vi "NeedRecalcPath.vi"(0 "Project":T1, 1 "AttackerAvoidArea":bool=TRUE, 4 "ignoreBall?":bool, 5 "Initial State":dbl[](array[numeric]), 6 "SmoothPath":dbl[][](array[numeric]), 7 "Pos x,y":dbl[](array[numeric]), 8 "Volta ao redor\nda área?":bool, 9 "IA State":T2={"our_robots"=[], "enemy_robots"=[], "balls"=[], "geometry"={"line_width"=0, "field_length"=0, "field_width"=0, "boundary_width"=0, "referee_width"=0, "goal_width"=0, "goal_depth"=0, "goal_wall_width"=0, "center_circle_radius"=0, "defense_radius"=0, "defense_stretch"=0, "free_kick_from_defense_dist"=0, "penalty_spot_from_field_line_dist"=0, "penalty_line_from_spot_dist"=0}, "IA Judge"={"stage"="", "command"="", "our_goalie_id"=0.0, "enemy_goalie_id"=0.0, "command enum"=enum."Halt", "Time"=enum."Azul", "Point"={"x"=0.0, "y"=0.0}}, "Received Timestamp"=timestamp(0 s since 1904-01-01), "Events"={"Touch"=FALSE, "Ball out"=FALSE, "id touch"=0.0, "Ball out of \nVision"=FALSE, "Ball inside \nGoalie area"=FALSE, "Robot not responding"=FALSE, "Robots responding status"=[1.0, 1.0, 1.0, 1.0, 1.0, 1.0], "Enemy Ball \nPossession"=FALSE, "Pass State"=FALSE, "id end of pass"=0.0, "Kick"=FALSE, "Id ini Possession"=0.0, "Ball Possesion"=FALSE, "Id Possesion"=0.0, "Direct Kick"=FALSE, "2nd Strk Ativo"=FALSE}}, 10 "Robot":T3={"id"=0, "function"=enum."Attacker", "x"=0.0, "y"=0.0, "orientation"=0.0, "v_tangent"=0.0, "v_normal"=0.0, "v_ang"=0.0, "kick_x"=0.0, "kick_z"=0.0, "dribble"=FALSE, "Timestamp"=timestamp(0 s since 1904-01-01), "estimatives"={"est_v_tangent"=0.0, "est_v_normal"=0.0, "est_vx"=0.0, "est_vy"=0.0, "Pos Robot Est"=[], "est_v_ang"=0.0}, "dest_x_kick"=0.0, "dest_y_kick"=0.0, "Gap Coord"=[], "States"=enum."Pass", "Path "=[], "Path  Smooth"=[], "Dest"=[], "vx_desired"=0.0, "vy_desired"=0.0, "slowBehavior"=FALSE, "VSSStates"=enum."Pass", "robotKickState"=enum."none", "role"=enum."DefenderArea", "x_k|k"=[], "driveMode"=enum."Fast"}, 11 "Dest x,y":dbl[](array[numeric])) -> (2 "result":bool, 3 "NeedRecalc":bool)   [LabVIEW 2023]
uses:
  Vision_class/Old vision/Controls/AI Robot.ctl
  Vision_class/Old vision/Controls/Functions Enum.ctl
  Controls/estimatives.ctl
  Vision_class/Old vision/Controls/AttackerStates.ctl
  Vision_class/Old vision/Controls/PathDests.ctl
  Vision_class/Old vision/Controls/PathDest.ctl
  Navigation/VSSNavigation/VSSAttackerStates.ctl
  Robot_class/robotKickToStates.ctl
  Robot_class/roles.ctl
  <vilib>/Analysis/Matrix/Datatypes/RealMatrix.ctl
  Navigation/driveMode.ctl
  Vision_class/Old vision/SSL Detection Frame Simple Estimator Cameras VelCmd Folder/Core/AI Input.ctl
  Vision_class/Old vision/SSL Detection Frame Simple Estimator Cameras VelCmd Folder/Core/AI Ball.ctl
  Vision_class/Old vision/SSL Detection Frame Simple Estimator Cameras VelCmd Folder/Core/Field Size.ctl
  Vision_class/Old vision/SSL Detection Frame Simple Estimator Cameras VelCmd Folder/Core/AI Judge.ctl
  Communication_class/Paths/MessageAI_State Folder/Intel/Command Enum.ctl
  Vision_class/Old vision/SSL Detection Frame Simple Estimator Cameras VelCmd Folder/Util/Events/Events.ctl
  Parameters_class/Project.ctl
  <vilib>/Analysis/_algsub.llb/Real Vector Norm.vi
  <vilib>/Analysis/NI_AALPro.lvlib
  <vilib>/Analysis/Matrix/NI_Matrix.lvlib
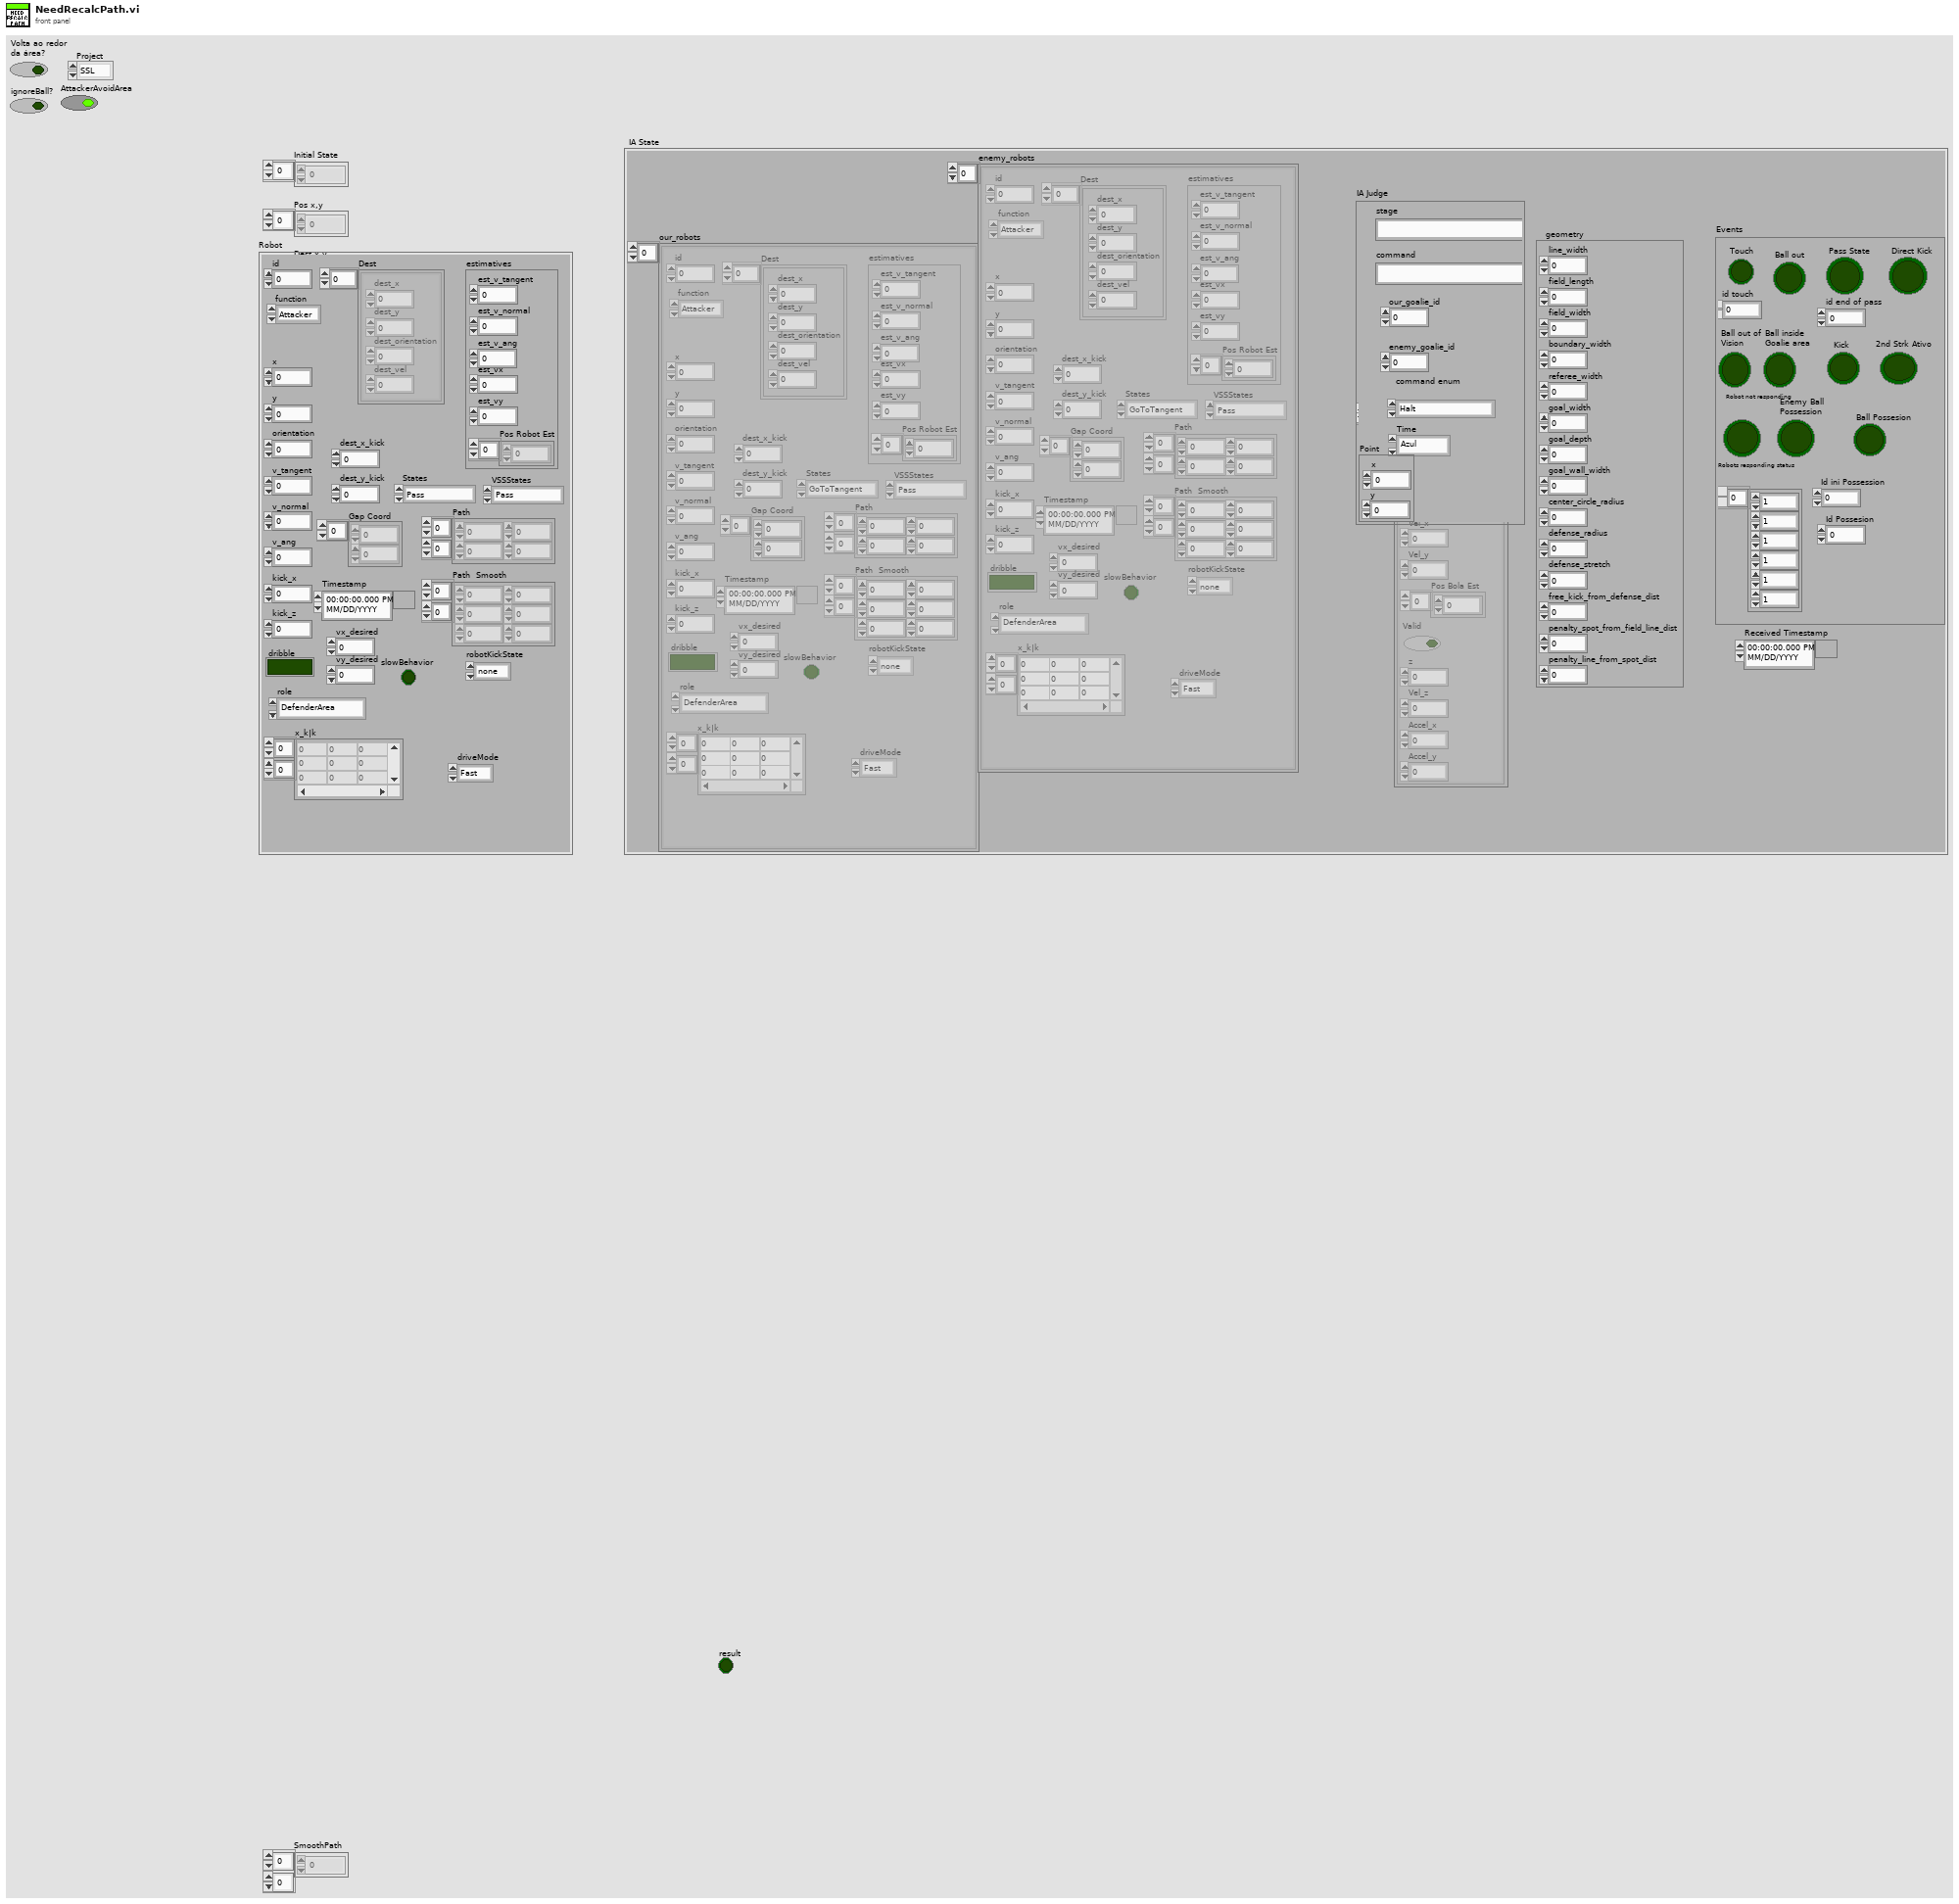
[diagram p1: front panel]
types:
  T1 = typedef "Project.ctl" = enum16{"SSL", "VSS"}
  T2 = typedef "AI Input.ctl" = cluster{"our_robots":T3[], "enemy_robots":T3[], "balls":T14[], "geometry":T15, "IA Judge":T16, "Received Timestamp":timestamp, "Events":T18}
  T3 = typedef "AI Robot.ctl" = cluster{"id":u32, "function":T4, "x":dbl, "y":dbl, "orientation":dbl, "v_tangent":dbl, "v_normal":dbl, "v_ang":dbl, "kick_x":dbl, "kick_z":dbl, "dribble":bool, "Timestamp":timestamp, "estimatives":T5, "dest_x_kick":dbl, "dest_y_kick":dbl, "Gap Coord":dbl[], "States":T6, "Path ":dbl[][], "Path  Smooth":dbl[][], "Dest":T7, "vx_desired":dbl, "vy_desired":dbl, "slowBehavior":bool, "VSSStates":T9, "robotKickState":T10, "role":T11, "x_k|k":T12, "driveMode":T13}
  T4 = typedef "Functions Enum.ctl" = enum16{"2nd Striker", "Attacker", "Goalie", "Defender", "Striker", "Goto 0", "Dummy", "Kicker", "ZigZag 0", "ZigZag 1", "ZigZag 2", "ZigZag 3", "ZigZag 4", "ZigZag 5", "ZigZag 6", "ZigZag 7", "ZigZag 8", ""}
  T5 = typedef "estimatives.ctl" = cluster{"est_v_tangent":dbl, "est_v_normal":dbl, "est_vx":dbl, "est_vy":dbl, "Pos Robot Est":dbl[], "est_v_ang":dbl}
  T6 = typedef "AttackerStates.ctl" = enum16{"Pass", "GoToTangent", "BallGetting", "GoToKick", ""}
  T7 = typedef "PathDests.ctl" = T8[]
  T8 = typedef "PathDest.ctl" = cluster{"dest_x":dbl, "dest_y":dbl, "dest_orientation":dbl, "dest_vel":dbl}
  T9 = typedef "VSSAttackerStates.ctl" = enum16{"Pass", "GoToTangent", "BallGetting", "GoToKick", "Rotate anti-clockwise", "Rotate Clockwise", ""}
  T10 = typedef "robotKickToStates.ctl" = enum16{"shootFromDirect", "avoidCollideBall", "goToBackBall", "none", "walk", "turn", "turnAntiClockWise", "turnClockwise", "oldKickToShoot", "oldKickToGoToBackBall", "shoot"}
  T11 = typedef "roles.ctl" = enum16{"SimpleBallPlacement", "BallPlacementAllyPasser", "BallPlacementAllyReceiver", "BallPlacementEnemy", "5Robots5th", "PassBestReceiver", "5Robots4th", "5Robots3rd", "5Robots2nd", "5Robots1st", "PassBestRobot", "WaitPass", "ABCThirdKicker", "ABCFirstKicker", "ABCSecondKicker", "Tabler", "TableFinalizer", "PrepareRollToPassRoller", "PrepareRollToPassReceiver", "SimplePassRoll", "SimplePassRollReceiver", "PenaltyDefense", "PreparePassReceiver 2", "PreparePassReceiver 1", "PassObserver", "Timeout", "Goto", "ZigZag", "None", "BallOutOfField", "DefenderArea", "Duelist", "AttackerStop", "FollowAttacker", "KeeperRole", "KickPenalty", "AttackerAimGoal", "AttackerBlock", "Marker", "Halt", "Shoot", "PassKicker", "PassReceiver", "TestRole", "PenaltyAttacker"}
  T12 = typedef "NI_Matrix.lvlib/RealMatrix.ctl" = dbl[][]
  T13 = typedef "driveMode.ctl" = enum16{"Fast", "SafeDrive"}
  T14 = typedef "AI Ball.ctl" = cluster{"x":dbl, "y":dbl, "timestamp":timestamp, "Vel_x":dbl, "Vel_y":dbl, "Pos Bola Est":dbl[], "Valid":bool, "z":dbl, "Vel_z":dbl, "Accel_x":dbl, "Accel_y":dbl}
  T15 = typedef "Field Size.ctl" = cluster{"line_width":u32, "field_length":u32, "field_width":u32, "boundary_width":u32, "referee_width":u32, "goal_width":u32, "goal_depth":u32, "goal_wall_width":u32, "center_circle_radius":u32, "defense_radius":u32, "defense_stretch":u32, "free_kick_from_defense_dist":u32, "penalty_spot_from_field_line_dist":u32, "penalty_line_from_spot_dist":u32}
  T16 = typedef "AI Judge.ctl" = cluster{"stage":string, "command":string, "our_goalie_id":dbl, "enemy_goalie_id":dbl, "command enum":T17, "Time":enum16{"Azul", "Amarelo"}, "Point":cluster{"x":sgl, "y":sgl}}
  T17 = typedef "Command Enum.ctl" = enum16{"Halt", "Stop", "Force Start", "PKA Normal Start", "Prepare Kickoff Ally", "PKE Normal Start", "Prepare Kickoff Enemy", "Prepare Penalty Ally", "PPA Normal Start", "Prepare Penalty Enemy", "PPE Normal Start", "Direct Free Enemy", "Direct Free Ally", "Indirect Free Enemy", "Indirect Free Ally", "Timeout Enemy", "Timeout Ally", "Goal Enemy", "Goal Ally", "Ball Placement Enemy", "Ball Placement Ally", "Normal Half Time", "Extra Time Break", "Extra Half Time", "None", "Post Game"}
  T18 = typedef "Events.ctl" = cluster{"Touch":bool, "Ball out":bool, "id touch":dbl, "Ball out of \nVision":bool, "Ball inside \nGoalie area":bool, "Robot not responding":bool, "Robots responding status":dbl[], "Enemy Ball \nPossession":bool, "Pass State":bool, "id end of pass":dbl, "Kick":bool, "Id ini Possession":dbl, "Ball Possesion":bool, "Id Possesion":dbl, "Direct Kick":bool, "2nd Strk Ativo":bool}
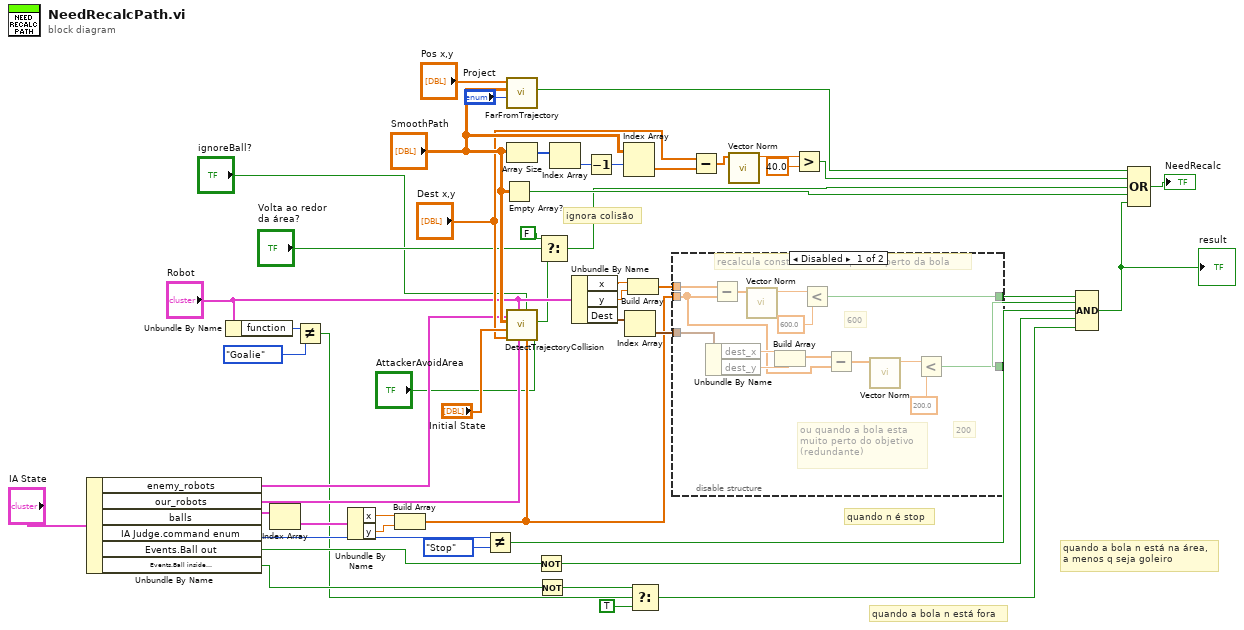
[diagram p0: block diagram]
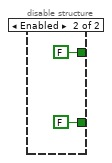
[diagram p2: hidden frame]
diagram:
  # "ignora colisão"
  # "quando a bola n está na área,\na menos q seja goleiro"
  # "quando n é stop"
  # "quando a bola n está fora"
  n1 = Unbundle By Name("IA State") -> ("enemy_robots"=w35:T3[], "our_robots"=w34:T3[], "balls"=w33:T14[], "IA Judge.command enum"=w23:T17, "Events.Ball out"=w18:bool, "Events.Ball inside \nGoalie area"=w13:bool)
  n2 = Unbundle By Name("Robot") -> ("function"=w20:T4)
  n3 = Index Array(array=w33) -> (element=w32:T14)  [unwired: 1 in]
  n4 = Not Equal?(x=w20, y=Functions_Enum."Goalie") -> (x != y?=w11:bool)
  n5 = Unbundle By Name(w32) -> ("x"=w28:dbl, "y"=w27:dbl)
  n6 = Build Array(w28, w27) -> (w24:dbl[])
  n7 = Not Equal?(x=w23, y=Command_Enum."Stop") -> (x != y?=w15:bool)
  n8 = Empty Array?(array="SmoothPath") -> (empty?=w46:bool)
  n9 = call "FarFromTrajectory.vi"("Project"="Project", "Path"="SmoothPath", "Position"="Pos x,y") -> ("Far from trajectory?"=w48:bool)  [unwired: 8 in]
  n10 = Array Size(array="SmoothPath") -> (size(s)=w37:i32[])
  n11 = call "DetectTrajectoryCollision.vi"("AttackerAvoidArea"="AttackerAvoidArea", "ball"=w24, "ignoreBall?"="ignoreBall?", "our_robots"=w34, "Robot in"="Robot", "Goal"="Dest x,y", "Initial State"="Initial State", "Last Path"="SmoothPath", "enemy_robots"=w35) -> ("Collision"=w6:bool)  [unwired: 2 in]
  n12 = Not(x=w18) -> (.not. x?=w14:bool)
  n13 = Not(x=w13) -> (.not. x?=w12:bool)
  n14 = Select(t=FALSE, s="Volta ao redor\nda área?", f=w6) -> (s? t:f=w5:bool)
  n15 = Index Array(array=w37) -> (element=w44:i32)  [unwired: 1 in]
  n16 = Unbundle By Name("Robot") -> ("x"=w31:dbl, "y"=w30:dbl, "Dest"=w26:T7)
  n17 = Decrement(x=w44) -> (x-1=w43:i32)
  n18 = Index Array(array="SmoothPath", index (row)=w43) -> (element=w38:dbl[])  [unwired: 1 in]
  n19 = Index Array(array=w26) -> (element=w25:T8)  [unwired: 1 in]
  n20 = Build Array(w31, w30) -> (w29:dbl[])
  n21 = Select(t=w12, s=w11, f=TRUE) -> (s? t:f=w9:bool)
  n22 = disable-structure shown="Disabled" {
    disable-tunnel: w29 -> [w65 _]
    disable-tunnel: w25 -> [w62 _]
    disable-tunnel: w24 -> [w54 _]
    disable-tunnel: [w53 FALSE] -> w16
    disable-tunnel: [w52 FALSE] -> w8
    frame Disabled {
      # "200"
      # "600"
      # "ou quando a bola esta\nmuito perto do objetivo\n(redundante)"
      # "recalcula constantemente quando perto da bola"
      n23 = Unbundle By Name(w62) -> ("dest_x"=w60:dbl, "dest_y"=w59:dbl)
      n24 = Subtract(x=w65, y=w54) -> (x-y=w64:dbl[])
      n25 = call-poly <vilib>:"Vector Norm.vi"("Input Vector"=w64) -> ("norm"=w63:dbl)  [unwired: 9 in, 1 out]
      n26 = Build Array(w60, w59) -> (w55:dbl[])
      n27 = Less?(x=w63, y=600.0) -> (x < y?=w52:bool)
      n28 = Subtract(x=w55, y=w54) -> (x-y=w56:dbl[])
      n29 = call-poly <vilib>:"Vector Norm.vi"("Input Vector"=w56) -> ("norm"=w57:dbl)  [unwired: 9 in, 1 out]
      n30 = Less?(x=w57, y=200.0) -> (x < y?=w53:bool)
    }
    frame Enabled {
    }
  }
  n31 = Subtract(x="Dest x,y", y=w38) -> (x-y=w39:dbl[])
  n32 = call-poly <vilib>:"Vector Norm.vi"("Input Vector"=w39) -> ("norm"=w40:dbl)  [unwired: 9 in, 1 out]
  n33 = Greater?(x=w40, y=40.0) -> (0:w41:bool)
  n34 = Compound Arithmetic op=AND(w8, w16, w15, w14, w9) -> (w17:bool)
  "result" <- w17
  n35 = Compound Arithmetic op=OR(w48, w41, w5, w46, w17) -> (→"NeedRecalc":bool)
